vi "Quick Drop.vi"(10 "Context":refnum<k7>, 11 "Engine":refnum<k7>) -> ()   [LabVIEW 2021, in "Seq Edit Quick Drop.lvlib"]
uses:
  Seq Edit Quick Drop.lvlib
  Command.ctl
  Data.ctl
  Message.ctl
  Register Item.ctl
  Connection Type.ctl
  Event Response.ctl
  <vilib>/Utility/SystemLogging/NI_SystemLogging.lvlib
  Dependencies/Tool Menu Utility.lvlibp/Tools/Tools.lvclass
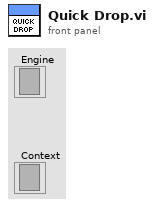
[diagram p1: front panel]
types:
  T1 = typedef "Seq Edit Quick Drop.lvlib/Message.ctl" = cluster{"cmd":T2, "data":variant}
  T2 = typedef "Seq Edit Quick Drop.lvlib/Command.ctl" = enum16{"Init", "Get Application Manager", "Shortcut Activated", "Display Tools", "Tool Selected", "Timeout", "Error", "Close"}
  T3 = typedef "Seq Edit Quick Drop.lvlib/Data.ctl" = cluster{"Engine":refnum<k7>, "Context":refnum<k7>, "Application Manager":refnum<k7>, "Register":map{string, T4}, "All Default Shortcuts":string[], "All Possible Shortcuts":string[], "Keys Mapping":map{string, string}}
  T4 = typedef "Seq Edit Quick Drop.lvlib/Register Item.ctl" = cluster{"Id":i32, "Path":string, "Events":refnum<k27>[]}
  T5 = typedef "Seq Edit Quick Drop.lvlib/Event Response.ctl" = cluster{"Connection Type":T6, "ID":i32}
  T6 = typedef "Seq Edit Quick Drop.lvlib/Connection Type.ctl" = enum16{"SequenceView", "SequenceList", "VariablesView"}
  T7 = cluster{"All Default Shortcuts":string[], "All Possible Shortcuts":string[], "Keys Mapping":map{string, string}}
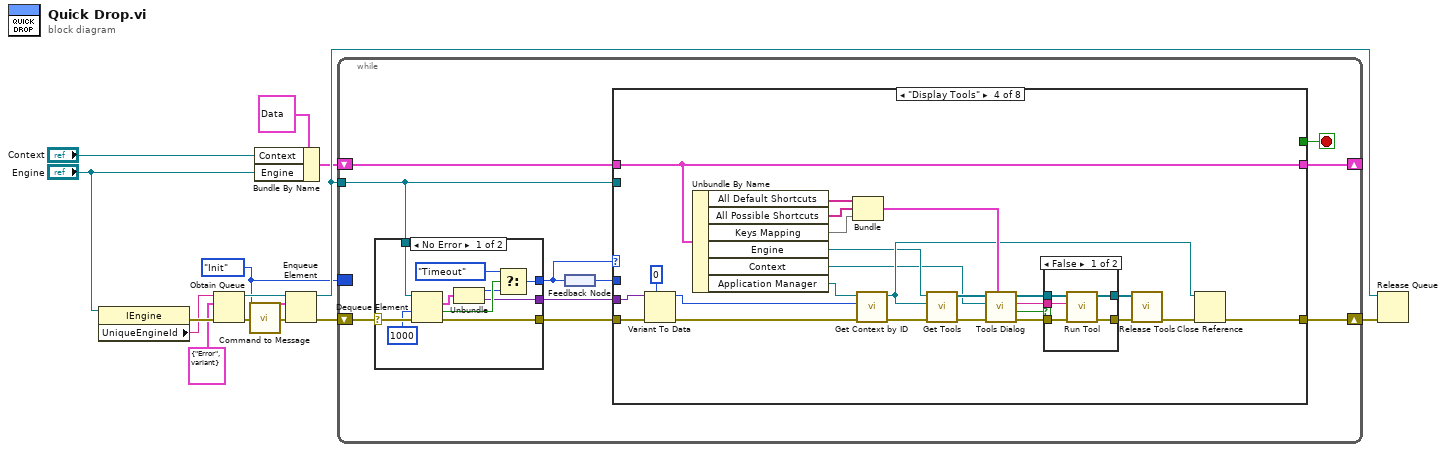
[diagram p0: block diagram]
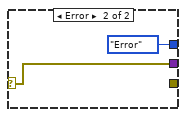
[diagram p2: hidden frame]
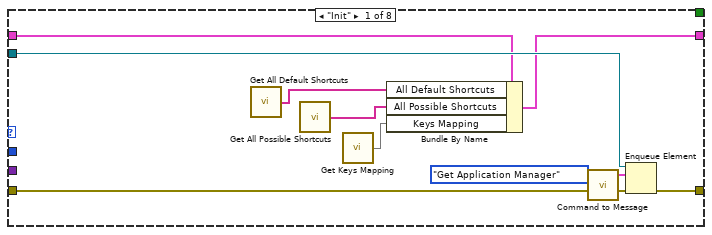
[diagram p3: hidden frame]
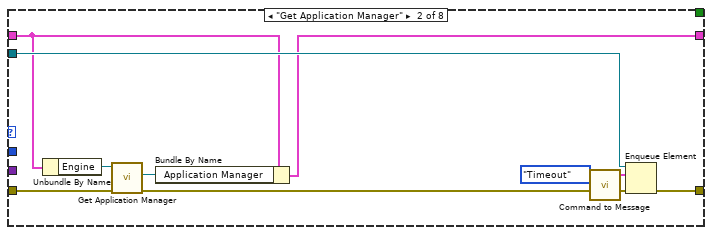
[diagram p4: hidden frame]
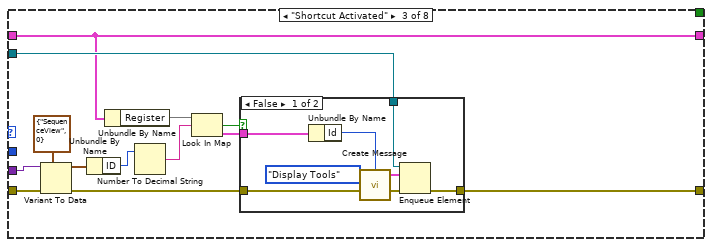
[diagram p5: hidden frame]
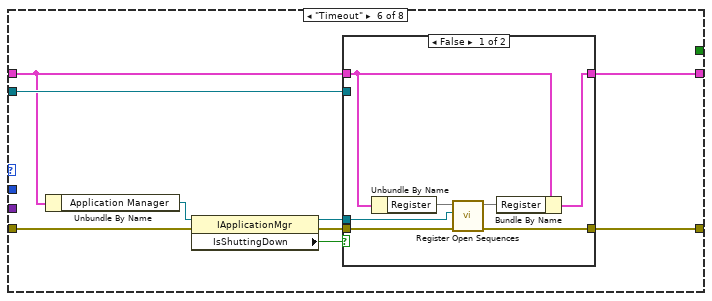
[diagram p9: hidden frame]
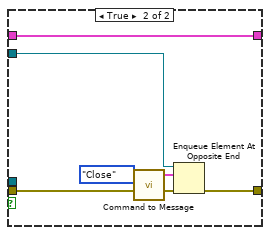
[diagram p10: hidden frame]
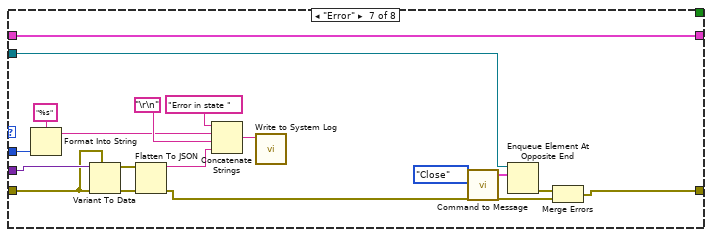
[diagram p11: hidden frame]
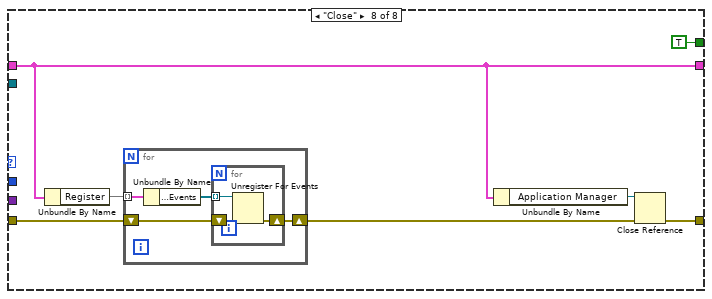
[diagram p12: hidden frame]
diagram:
  w3 = Command."Init" ("cmd")
  n1 = property class="IEngine"(reference="Engine") -> (error out=w13:errorcluster, "UniqueEngineId"=w7:string)  [unwired: 1 in, 1 out]
  n2 = Obtain Queue(name (unnamed)=w7, element data type=T1 {"cmd"=enum."Error", "data"=variant} ("cmd"), error in (no error)=w13) -> (queue out=w6:refnum<queue>, error out=w5:errorcluster)  [unwired: 2 in, 1 out]
  n3 = call "Command to Message.vi"("cmd"=w3) -> ("msg"=w2:T1)  [unwired: 4 in]
  n4 = Bundle By Name(cluster=T3 {"Engine"=refnum, "Context"=refnum, "Application Manager"=refnum, "Register"={}, "All Default Shortcuts"=[], "All Possible Shortcuts"=[], "Keys Mapping"={}} ("Data"), "Context"="Context", "Engine"="Engine") -> (w10:T3)
  n5 = Enqueue Element(queue=w6, element=w2, error in (no error)=w5) -> (queue out=w14:refnum<queue>, error out=w4:errorcluster)  [unwired: 1 in, 1 out]
  n6 = while {
    border: w3 -> [_]
    shift-right: [w19] -> w12
    shift-left: w4 -> [w23]
    shift-right: [w16] -> _
    shift-left: w10 -> [w17]
    tunnel: w14 -> [w15]
    stop <- w18 stop-if-true
    n7 = case shown="No Error" w23 {
      selector: w23 -> [w34 w35]
      tunnel: [w31 Command."Error" ("cmd")] -> w20
      tunnel: [w33 _] -> w22
      tunnel: [w25 w35] -> w21
      tunnel: w15 -> [w28 _]
      frame No Error {
        n8 = Dequeue Element(queue=w28, timeout in ms (-1)=1000, error in (no error)=w34) -> (element=w27:T1, timed out?=w32:bool, error out=w33:errorcluster)  [unwired: 1 out]
        n9 = Unbundle(w27) -> ("cmd"=w26:T2, "data"=w25:variant)
        n10 = Select(t=Command."Timeout", s=w32, f=w26) -> (s? t:f=w31:T2)
      }
      frame Error {
      }
    }
    n11 = feedback #1() -> (w24:T2)
    n12 = feedback-in #1(w20) -> ()
    n13 = case shown="\"Display Tools\"" w20 {
      tunnel: w24 -> [_ _ _ _ _ _ w139 _]
      tunnel: w22 -> [w46 w55 w68 w101 w111 w119 w142 w154]
      tunnel: w21 -> [_ _ w67 w99 _ _ w143 _]
      tunnel: [w45 w53 w57 w95 w111 w116 w135 w158] -> w19
      tunnel: [_ _ _ _ _ _ _ TRUE] -> w18
      tunnel: w17 -> [w37 w52 w63 w96 w110 w112 w150 w155]
      tunnel: [w38 w50 w63 w96 w110 w113 w150 w155] -> w16
      tunnel: w15 -> [w44 w56 w69 _ _ w120 w149 _]
      frame "Init" {
        n14 = call "Get All Default Shortcuts.vi"() -> ("All Default Shortcuts"=w41:string[])
        n15 = call "Get All Possible Shortcuts.vi"() -> ("All Possible Shortcuts"=w40:string[])
        n16 = call "Get Keys Mapping.vi"() -> ("Keys Mapping"=w39:map{string, string})
        n17 = Bundle By Name(cluster=w37, "All Default Shortcuts"=w41, "All Possible Shortcuts"=w40, "Keys Mapping"=w39) -> (w38:T3)
        n18 = call "Command to Message.vi"("cmd"=Command."Get Application Manager") -> ("msg"=w43:T1)  [unwired: 4 in]
        n19 = Enqueue Element(queue=w44, element=w43, error in (no error)=w46) -> (error out=w45:errorcluster)  [unwired: 1 in, 2 out]
      }
      frame "Get Application Manager" {
        n20 = Unbundle By Name(w52) -> ("Engine"=w51:refnum<k7>)
        n21 = call "Get Application Manager.vi"("Error In"=w55, "Engine In"=w51) -> ("Error Out"=w54:errorcluster, "Application Manager"=w49:refnum<k7>)  [unwired: 7 in, 1 out]
        n22 = Bundle By Name(cluster=w52, "Application Manager"=w49) -> (w50:T3)
        n23 = call "Command to Message.vi"("cmd"=Command."Timeout") -> ("msg"=w47:T1)  [unwired: 4 in]
        n24 = Enqueue Element(queue=w56, element=w47, error in (no error)=w54) -> (error out=w53:errorcluster)  [unwired: 1 in, 2 out]
      }
      frame "Shortcut Activated" {
        n25 = Variant To Data(error in=w68, type=T5 {"Connection Type"=enum."SequenceView", "ID"=0} ("Event Response"), Variant=w67) -> (data=w65:T5, error out=w58:errorcluster)
        n26 = Unbundle By Name(w65) -> ("ID"=w64:i32)
        n27 = Unbundle By Name(w63) -> ("Register"=w62:map{string, T4})
        n28 = Number To Decimal String(number=w64) -> (decimal integer string=w61:string)  [unwired: 1 in]
        n29 = Look In Map(map=w62, key=w61) -> (key not found?=w59:bool, value=w60:T4)  [unwired: 1 in]
        n30 = case shown="False" w59 {
          tunnel: w60 -> [w76 _]
          tunnel: w58 -> [w75 w77]
          tunnel: [w74 w77] -> w57
          tunnel: w69 -> [w73 _]
          frame False {
            n31 = Unbundle By Name(w76) -> ("Id"=w71:i32)
            n32 = call "Create Message.vi"("cmd"=Command."Display Tools", "data"=w71) -> ("msg"=w72:T1)  [unwired: 2 in]
            n33 = Enqueue Element(queue=w73, element=w72, error in (no error)=w75) -> (error out=w74:errorcluster)  [unwired: 1 in, 2 out]
          }
          frame True {
          }
        }
      }
      frame "Display Tools" {
        n34 = Variant To Data(error in=w101, type=0, Variant=w99) -> (data=w97:i32, error out=w100:errorcluster)
        n35 = Unbundle By Name(w96) -> ("All Default Shortcuts"=w82:string[], "All Possible Shortcuts"=w81:string[], "Keys Mapping"=w80:map{string, string}, "Engine"=w89:refnum<k7>, "Context"=w78:refnum<k7>, "Application Manager"=w79:refnum<k7>)
        n36 = Bundle("All Default Shortcuts"=w82, "All Possible Shortcuts"=w81, "Keys Mapping"=w80) -> (w102:T7)  [unwired: 1 in]
        n37 = call "Get Context by ID.vi"("Error In"=w100, "Sequence ID"=w97, "Application Manager"=w79) -> ("Error Out"=w92:errorcluster, "Sequence Context"=w90:refnum<k7>)  [unwired: 7 in]
        n38 = call "Get Tools.vi"("Error In"=w92, "Context"=w90, "Engine"=w89) -> ("Error Out"=w91:errorcluster, "Tools"=w88:refnum<class "Tools.lvclass">[])  [unwired: 7 in]
        n39 = call "Tools Dialog.vi"("Settings"=w102, "Error In"=w91, "Context"=w78, "Tools In"=w88) -> ("Error Out"=w94:errorcluster, "Canceled?"=w84:bool, "ID"=w86:string, "Tools Out"=w85:refnum<class "Tools.lvclass">[])  [unwired: 4 in]
        n40 = case shown="False" w84 {
          tunnel: w94 -> [w107 w109]
          tunnel: [w106 w109] -> w93
          tunnel: w86 -> [w105 _]
          tunnel: w85 -> [w104 w108]
          tunnel: [w103 w108] -> w83
          frame False {
            n41 = call "Run Tool.vi"("Error In"=w107, "ID"=w105, "Tools In"=w104) -> ("Error Out"=w106:errorcluster, "Tools Out"=w103:refnum<class "Tools.lvclass">[])  [unwired: 7 in]
          }
          frame True {
          }
        }
        n42 = call "Release Tools.vi"("Error In"=w93, "Tools"=w83) -> ("Error Out"=w87:errorcluster)  [unwired: 9 in]
        n43 = Close Reference(reference=w90, error in (no error)=w87) -> (error out=w95:errorcluster)
      }
      frame "Tool Selected" {
        # "Placeholder case for executing super quick shorcuts"
        # "#TODO"
      }
      frame "Timeout" {
        n44 = Unbundle By Name(w112) -> ("Application Manager"=w115:refnum<k7>)
        n45 = property class="IApplicationMgr"(reference=w115, error in=w119) -> (reference out=w114:refnum<k7>, error out=w117:errorcluster, "IsShuttingDown"=w118:bool)
        n46 = case shown="False" w118 {
          tunnel: w117 -> [w127 w133]
          tunnel: [w126 w132] -> w116
          tunnel: w120 -> [_ w131]
          tunnel: w114 -> [w125 _]
          tunnel: w112 -> [w123 w128]
          tunnel: [w121 w128] -> w113
          frame False {
            n47 = Unbundle By Name(w123) -> ("Register"=w124:map{string, T4})
            n48 = call "Register Open Sequences.vi"("Error In"=w127, "Application Manager In"=w125, "Register In"=w124) -> ("Error Out"=w126:errorcluster, "Register Out"=w122:map{string, T4})  [unwired: 7 in]
            n49 = Bundle By Name(cluster=w123, "Register"=w122) -> (w121:T3)
          }
          frame True {
            n50 = call "Command to Message.vi"("cmd"=Command."Close") -> ("msg"=w129:T1)  [unwired: 4 in]
            n51 = Enqueue Element At Opposite End(queue=w131, element=w129, error in (no error)=w133) -> (error out=w132:errorcluster)  [unwired: 1 in, 2 out]
          }
        }
      }
      frame "Error" {
        n52 = Format Into String(format string="%s", w139) -> (resulting string=w138:string)  [unwired: 2 in, 1 out]
        n53 = Variant To Data(error in=w142, type=w142, Variant=w143) -> (data=w141:errorcluster, error out=w140:errorcluster)
        n54 = Flatten To JSON(anything=w141, error in (no error)=w140) -> (JSON string=w137:string, 11:w134:errorcluster)  [unwired: 1 in]
        n55 = Concatenate Strings("Error in state " ("string"), w138, "\r\n", w137) -> (w145:string)
        n56 = call <vilib>:"Write to System Log.vi"("message"=w145) -> ()  [unwired: 10 in, 1 out]
        n57 = call "Command to Message.vi"("cmd"=Command."Close") -> ("msg"=w147:T1)  [unwired: 4 in]
        n58 = Enqueue Element At Opposite End(queue=w149, element=w147) -> (error out=w151:errorcluster)  [unwired: 2 in, 2 out]
        n59 = Merge Errors(w151, w134) -> (w135:errorcluster)
      }
      frame "Close" {
        n60 = Unbundle By Name(w155) -> ("Register"=w153:map{string, T4})
        n61 = for {
          shift-right: [w162] -> w152
          shift-left: w154 -> [w161]
          tunnel: w153 -> [w160] mode=indexing
          n62 = Unbundle By Name(w160) -> ("Register Item.Events"=w159:refnum<k27>[])
          n63 = for {
            tunnel: w159 -> [w163] mode=indexing
            shift-right: [w165] -> w162
            shift-left: w161 -> [w164]
            n64 = Unregister For Events(event registration refnum=w163, error in=w164) -> (error out=w165:errorcluster)
          }
        }
        n65 = Unbundle By Name(w155) -> ("Application Manager"=w157:refnum<k7>)
        n66 = Close Reference(reference=w157, error in (no error)=w152) -> (error out=w158:errorcluster)
      }
    }
  }
  n67 = Release Queue(queue=w14, error in (no error)=w12) -> ()  [unwired: 1 in, 3 out]
